vi "FFT+wfm.vi"() -> ()   [LabVIEW 2020]
uses:
  <vilib>/Analysis/2dsp.llb/Real FFT.vi
  <vilib>/Instr/_visa.llb/VISA Configure Serial Port (Instr).vi
  <vilib>/Analysis/NI_AALPro.lvlib
panel:
  in  "stop 2":bool
  out "String":string
  out "data out":string
  out "bytes written":i32
  out "max i":i32
  in  "VISA resource name":refnum<visa-resource-name>
  out "XY Graph":cluster{dbl[], dbl[]}(graph)
  out "r":dbl[](array[numeric])
  out "size(s)":i32
  out "Waveform Chart":i32[](graph)
  in  "stop":bool
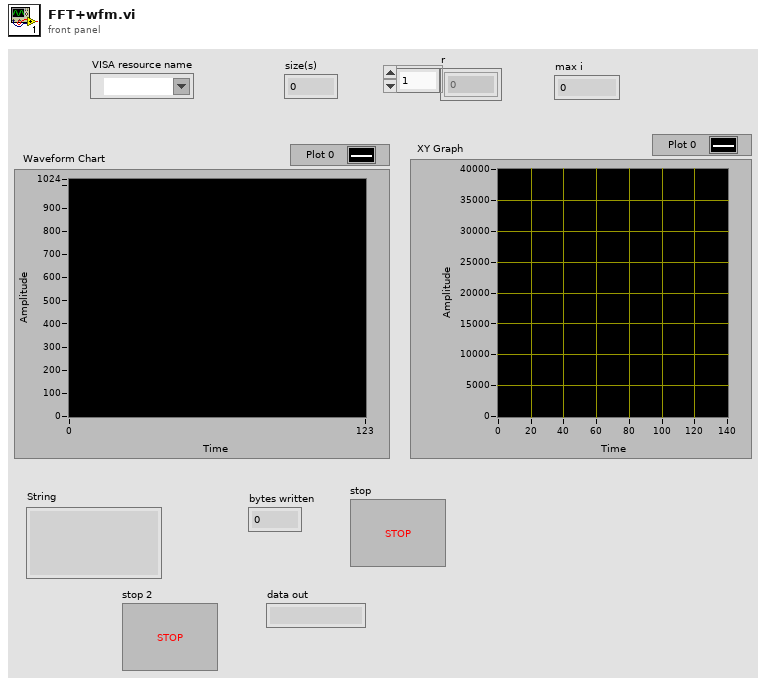
[diagram p1: front panel]
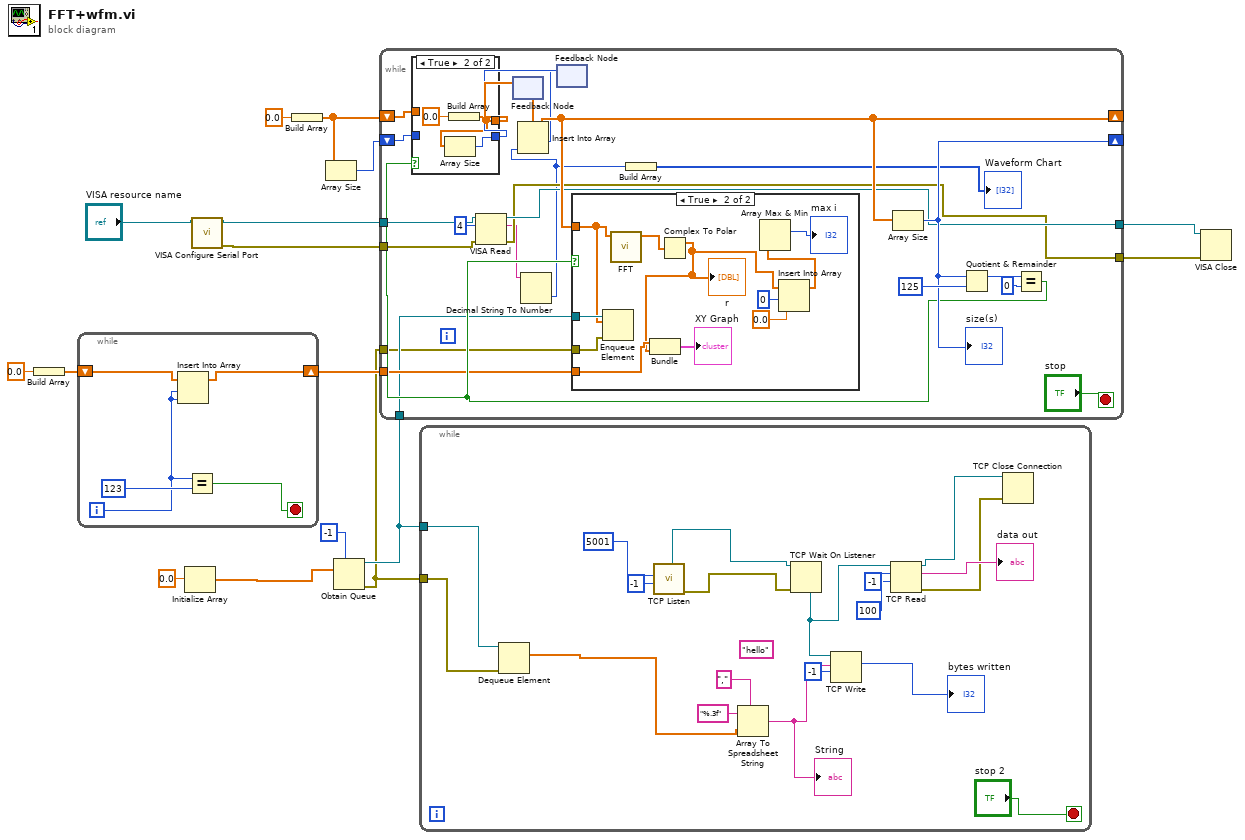
[diagram p0: block diagram]
diagram:
  n1 = Build Array(0.0 ("element")) -> (w13:dbl[])
  n2 = while {
    shift-right: [w20] -> w11
    shift-left: w13 -> [w21]
    i -> [w18]
    stop <- w17 stop-if-true
    n3 = Insert Into Array(array=w21, index=w18, new element=w18) -> (w20:dbl[])
    n4 = Equal?(x=w18, y=123) -> (x = y?=w17:bool)
  }
  n5 = Initialize Array(0.0) -> (w3:dbl[])  [unwired: 1 in]
  n6 = call-poly "VISA Configure Serial Port"("VISA resource name"="VISA resource name") -> ("VISA resource name out"=w7:refnum<visa-resource-name>, "error out"=w6:errorcluster)  [unwired: 13 in]
  n7 = Build Array(0.0 ("element")) -> (w14:dbl[])
  n8 = Array Size(array=w14) -> (size(s)=w15:i32)
  n9 = Obtain Queue(max queue size (-1, unlimited)=-1, element data type=w3) -> (queue out=w2:refnum<queue>, error out=w1:errorcluster)  [unwired: 3 in, 1 out]
  n10 = while {
    shift-right: [w40] -> _
    shift-left: w15 -> [w39]
    shift-right: [w44] -> _
    shift-left: w14 -> [w38]
    tunnel: w11 -> [w32]
    tunnel: w7 -> [w31]
    tunnel: w6 -> [w30]
    tunnel: [w29] -> w10
    tunnel: [w28] -> w9
    tunnel: w2 -> [w23]
    tunnel: w1 -> [w22]
    stop <- "stop" stop-if-true
    n11 = VISA Read(VISA resource name=w31, byte count=u32 4, error in (no error)=w30) -> (VISA resource name out=w29:refnum<visa-resource-name>, read buffer=w27:string, error out=w28:errorcluster)  [unwired: 1 out]
    n12 = feedback #1() -> (w35:dbl[])  [unwired: 1 in]
    n13 = Decimal String To Number(string=w27) -> (number=w25:i32)  [unwired: 2 in, 1 out]
    n14 = feedback #2() -> (w33:i32)  [unwired: 1 in]
    n15 = Insert Into Array(array=w35, index=w33, new element=w25) -> (w44:dbl[])
    n16 = Build Array(w25) -> (→"Waveform Chart":i32[])
    n17 = Array Size(array=w44) -> (size(s)=w40:i32)
    "size(s)" <- w40
    n18 = Quotient & Remainder(x=w40, y=125) -> (x-y*floor(x/y)=w42:i32)  [unwired: 1 out]
    n19 = Equal?(x=w42, y=0) -> (x = y?=w37:bool)
    n20 = case shown="True" w37 {
      tunnel: w39 -> [w46 _]
      tunnel: w38 -> [w47 _]
      tunnel: [w47 w48] -> w36
      tunnel: [w46 w49] -> w34
      frame False {
      }
      frame True {
        n21 = Build Array(0.0 ("element")) -> (w48:dbl[])
        n22 = Array Size(array=w48) -> (size(s)=w49:i32)
      }
    }
    n23 = feedback-in #1(w36) -> ()
    n24 = feedback-in #2(w34) -> ()
    n25 = case shown="True" w37 {
      tunnel: w44 -> [_ w51]
      tunnel: w32 -> [_ w60]
      tunnel: w23 -> [_ w53]
      tunnel: w22 -> [_ w52]
      frame False {
      }
      frame True {
        n26 = Enqueue Element(queue=w53, element=w51, error in (no error)=w52) -> ()  [unwired: 1 in, 3 out]
        n27 = call-poly <vilib>:"FFT.vi"("X"=w51) -> ("FFT {X}"=w61:cdb[])  [unwired: 9 in, 1 out]
        n28 = Complex To Polar(r * e^(i*theta)=w61) -> (r=w55:dbl[])  [unwired: 1 out]
        "r" <- w55
        n29 = Bundle(w60, w55) -> (→"XY Graph":cluster{dbl[], dbl[]})  [unwired: 1 in]
        n30 = Insert Into Array(array=w55, index=0, new element=0.0 ("new element/subarray")) -> (w54:dbl[])
        n31 = Array Max & Min(array=w54) -> (max index (indices)=→"max i":i32)  [unwired: 3 out]
      }
    }
  }
  n32 = while {
    tunnel: w2 -> [w64]
    tunnel: w1 -> [w63]
    stop <- "stop 2" stop-if-true
    (unwired) "hello" ("data in")
    n33 = Dequeue Element(queue=w64, error in (no error)=w63) -> (element=w62:dbl[])  [unwired: 1 in, 3 out]
    n34 = call <vilib>:"TCP Listen.vi"("timeout ms (wait forever: -1)"=-1, "port"=u16 5001) -> ("error out"=w71:errorcluster, "listener ID"=w73:refnum<k5>)  [unwired: 5 in, 3 out]
    n35 = Array To Spreadsheet String(delimiter (Tab)=",", array=w62, 3:"%.3f" ("format string")) -> (spreadsheet string=w69:string)
    "String" <- w69
    n36 = TCP Wait On Listener(8:w71, 11:w73) -> (4:w72:refnum<k5>)  [unwired: 2 in, 4 out]
    n37 = TCP Write(connection ID=w72, data in=w69, 9:-1 ("timeout ms (25000)")) -> (bytes written=→"bytes written":i32)  [unwired: 1 in, 2 out]
    n38 = TCP Read(connection ID=w72, bytes to read=100, 9:-1 ("timeout ms (25000)")) -> (connection ID out=w68:refnum<k5>, data out=→"data out":string, error out=w67:errorcluster)  [unwired: 2 in]
    n39 = TCP Close Connection(connection ID=w68, error in (no error)=w67) -> ()  [unwired: 1 in, 2 out]
  }
  n40 = VISA Close(VISA resource name=w10, error in (no error)=w9) -> ()  [unwired: 1 out]
